vi "ExReadFileHeaderPixRes.vi"(5 "error in (no error)":errorcluster) -> (4 "error out":errorcluster)   [LabVIEW 2010]
panel:
  in  "Full File Name":path
  in  "FileType":u32=67174400
  out "Pixel Y Resolution":u32
  out "Pixel X Resolution":u32
  # "ExReadSpeFileHeaderPixRes.vi\nThis VI will use read pixel resolution information stored in the file header\nand display it."
  # "File Types:\nSPE = 67371008\nTIF  = 67174400\nPMI = 67436544"
  # "Browse match pattern is set to *.tif.  Modify this if different file type is needed."
  # "um"
  # "um"
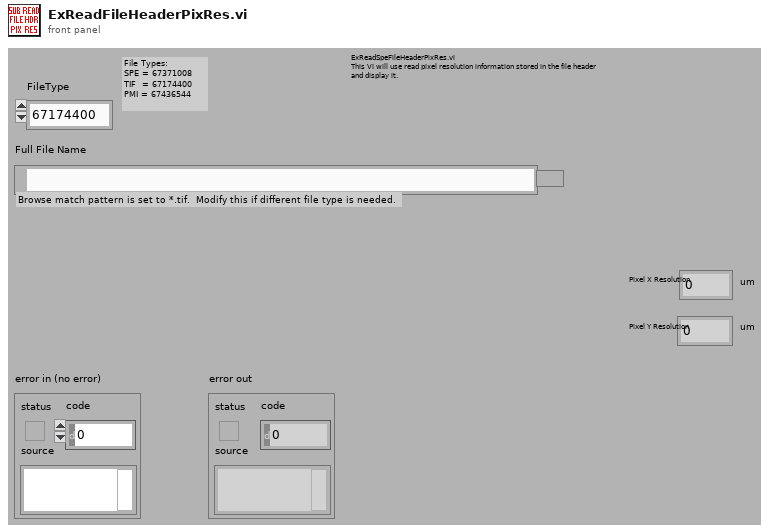
[diagram p1: front panel]
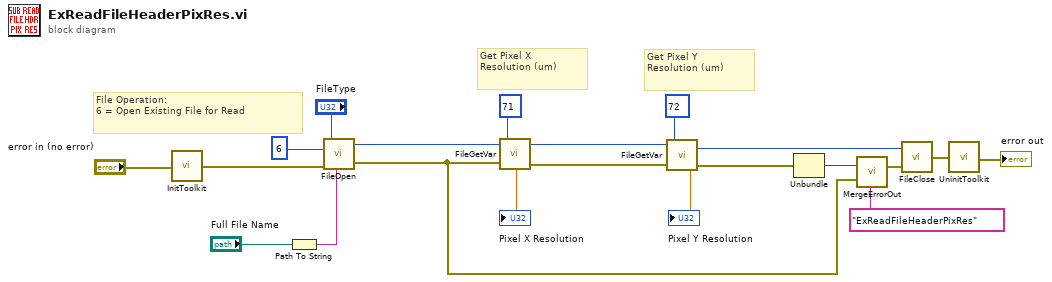
[diagram p0: block diagram]
diagram:
  # "File Operation:\n6 = Open Existing File for Read"
  # "Get Pixel Y\nResolution (um)"
  # "Get Pixel X\nResolution (um)"
  n1 = call <userlib>:"InitToolkit.vi"("error in"="error in (no error)") -> ("error out"=w14:errorcluster)
  n2 = Path To String(path="Full File Name") -> (string=w13:string)
  n3 = call <userlib>:"FileOpen.vi"("error in"=w14, "File Operations"=u32 6 ("File Operation"), "FileName"=w13, "File Type"="FileType") -> ("error out"=w3:errorcluster, "File Handle"=w4:u32)
  n4 = call <userlib>:"FileGetVar.vi"("error in"=w3, "Parameter ID"=71, "File Handle"=w4) -> ("error out"=w18:errorcluster, "Value"=→"Pixel X Resolution":dbl, "File Handle"=w19:u32)
  n5 = call <userlib>:"FileGetVar.vi"("error in"=w18, "Parameter ID"=72, "File Handle"=w19) -> ("error out"=w1:errorcluster, "Value"=→"Pixel Y Resolution":dbl, "File Handle"=w5:u32)
  n6 = Unbundle(w1) -> ("code"=w7:i32)  [unwired: 2 out]
  n7 = call <userlib>:"MergeErrorOut.vi"("error in"=w3, "Fucntion Name"="ExReadFileHeaderPixRes", "ErrorCode"=w7) -> ("error out"=w9:errorcluster)
  n8 = call <userlib>:"FileClose.vi"("error in"=w9, "File Handle"=w5) -> ("error out"=w6:errorcluster)
  n9 = call <userlib>:"UninitToolkit.vi"("error in"=w6) -> ("error out"=→"error out":errorcluster)
